vi "Framework Page.vi"(8 "error in (no error)":errorcluster, 11 "Node Ptr":T1 format="%.0x") -> (0 "error out":errorcluster)   [LabVIEW 2017, in "DSF System Explorer.lvlib"]
uses:
  DSF System Explorer.lvlib
  <vilib>/NI Veristand/Custom Device API/Custom Device Item Ref.ctl
  <vilib>/NI Veristand/Custom Device API/Custom Device API.lvlib
  Shared/DSF Shared.lvlib
panel:
  in  "Launch Data Viewer":bool
  in  "Server Frequency":dbl=20.0 format="%.0f Hz"
  in  "Enable Data Server":bool
  in  "Show Dialog on Error":bool
  in  "Show Threads":bool
  in  "Infinite FIFO Timeouts":bool
  in  "Measure Durations":bool
  in  "Measure Period":bool
  in  "Refresh Configuration":bool
  in  "View Configuration":bool
  in  "DSF Configuration Path":path
  in  "Header":cluster{"Section Name":string}={"Section Name"="Data Sharing Framework"}
  # "Debug Options"
  # "Measurement Options"
  # "Data Server Options"
  # "All Targets"
  # "All Targets"
  # "All Targets"
  # "Windows Only"
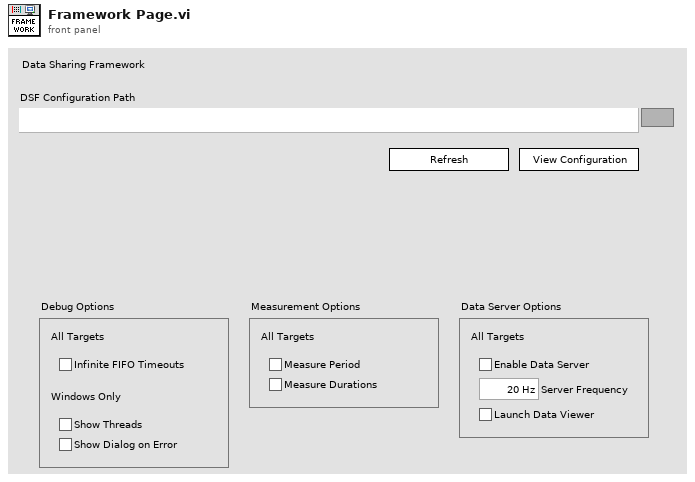
[diagram p1: front panel]
types:
  T1 = typedef "Custom Device API.lvlib/Custom Device Item Ref.ctl" = u64
  T2 = typedef "DSF Core.lvlibp/Framework.lvclass/Framework Options.ctl" = cluster{"FIFO Options":T3, "Thread Options":T4, "Plugin Options":T5, "Performance Options":T6, "Data Server Options":T7}
  T3 = typedef "DSF Core.lvlibp/Framework.lvclass/DSF FIFO Options.ctl" = cluster{"Infinite Timeouts":bool}
  T4 = typedef "DSF Core.lvlibp/Thread.lvclass/Thread Options.ctl" = cluster{"Show FP On Call":bool, "Close FP After Call":bool, "Allow Debugging":bool}
  T5 = typedef "DSF Core.lvlibp/Framework.lvclass/DSF Plugin Options.ctl" = cluster{"Default Components":bool}
  T6 = typedef "DSF Core.lvlibp/DSF Performance Options.ctl" = cluster{"Measure Period":bool, "Measure Rx/Tx Duration":bool}
  T7 = typedef "DSF Core.lvlibp/Framework.lvclass/Data Server Options.ctl" = cluster{"Enable Data Server":bool, "Period":u32}
  T8 = typedef "Custom Device API.lvlib/Custom Device Commands.ctl" = enum16{"Default", "Item renamed", "Shutdown", "Dynamic button pressed"}
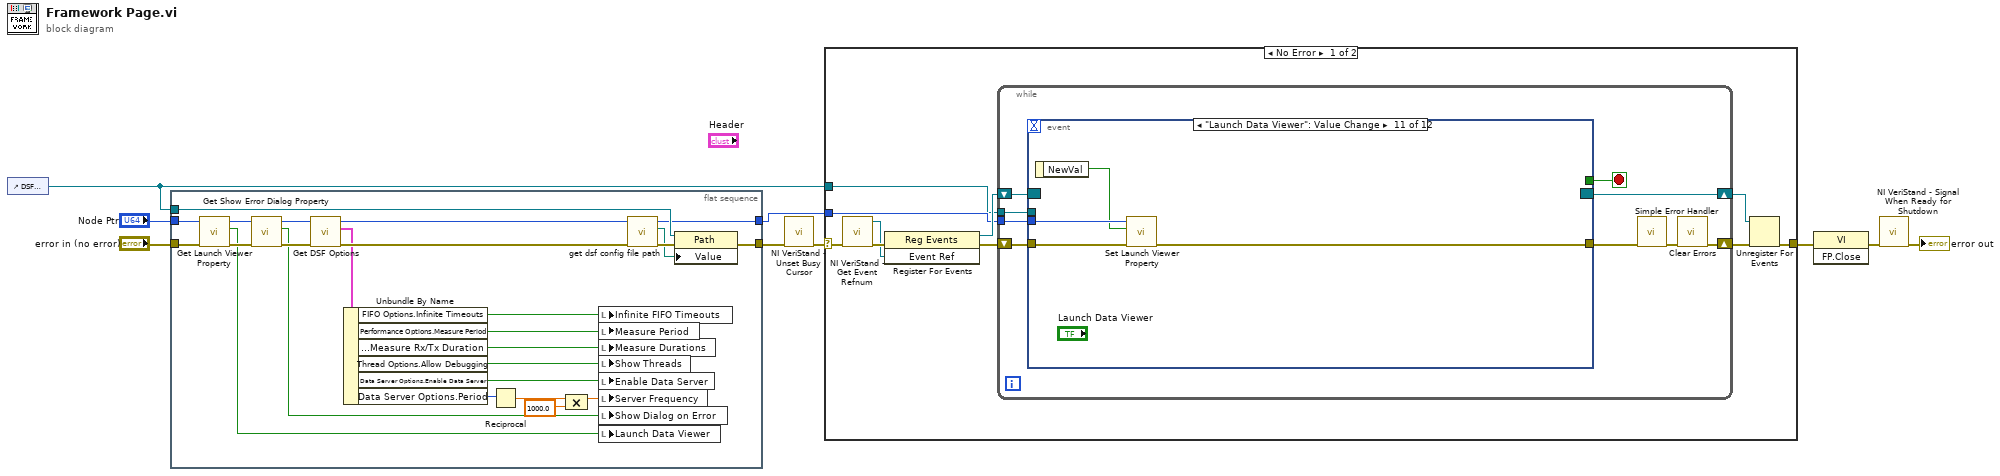
[diagram p0: block diagram]
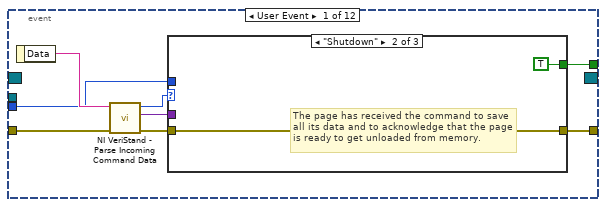
[diagram p2: hidden frame]
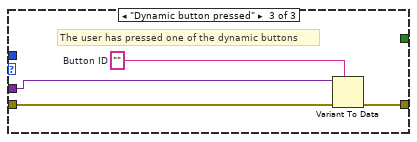
[diagram p4: hidden frame]
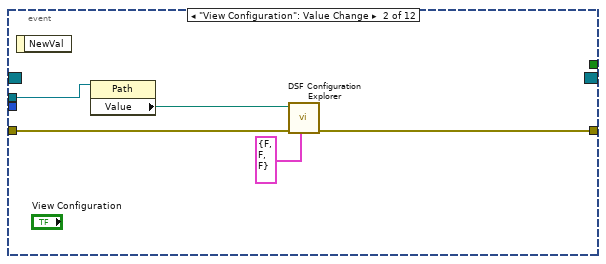
[diagram p5: hidden frame]
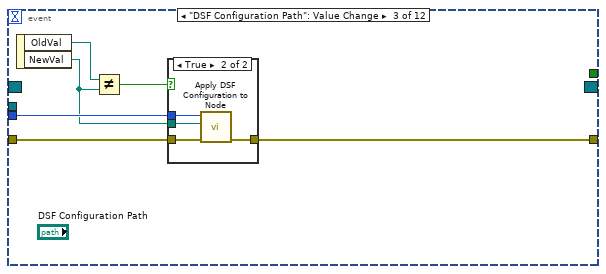
[diagram p6: hidden frame]
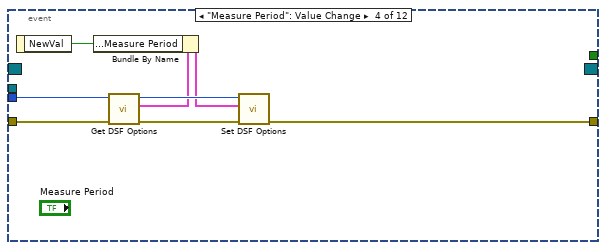
[diagram p8: hidden frame]
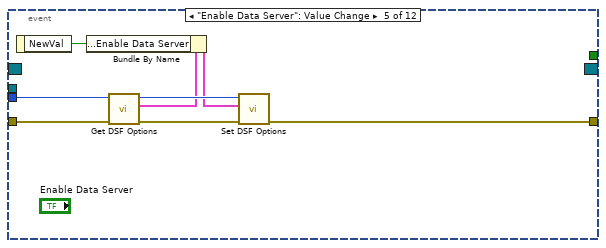
[diagram p9: hidden frame]
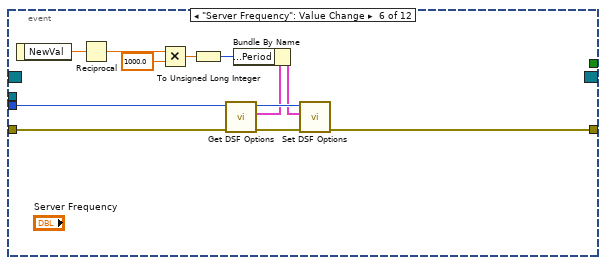
[diagram p10: hidden frame]
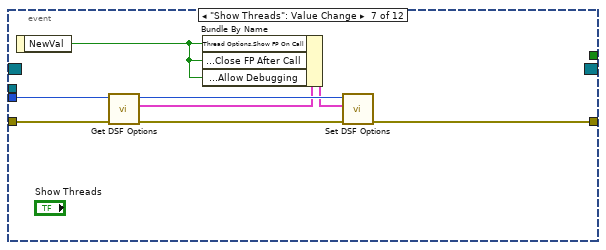
[diagram p11: hidden frame]
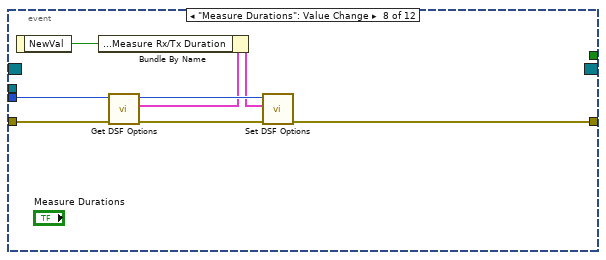
[diagram p12: hidden frame]
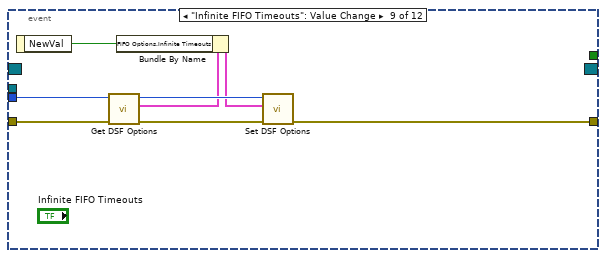
[diagram p13: hidden frame]
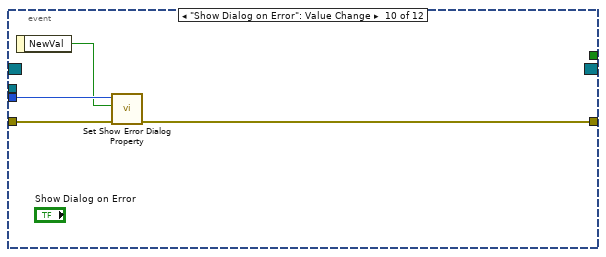
[diagram p14: hidden frame]
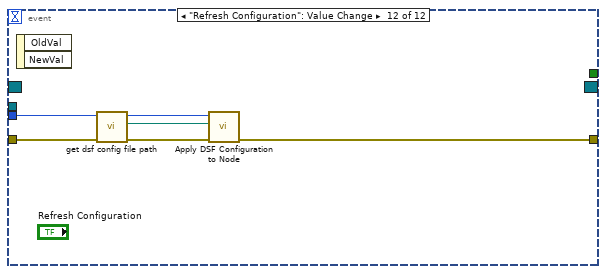
[diagram p15: hidden frame]
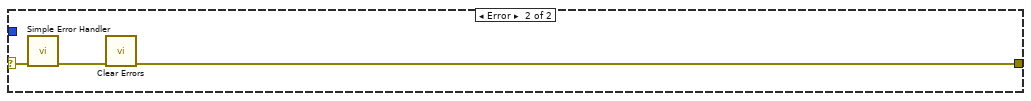
[diagram p16: hidden frame]
diagram:
  n1 = control-ref of="DSF Configuration Path"() -> (w1:refnum<vi>)
  n2 = flat-sequence "Initialization code" {
    tunnel: "error in (no error)" -> [w14]
    tunnel: "Node Ptr" -> [w13]
    tunnel: [w33] -> w5
    tunnel: [w31] -> w2
    tunnel: w1 -> [w32]
    frame #0 {
      n3 = call "Get Launch Viewer Property.vi"("error in (no error)"=w14, "Item Ref in"=w13) -> ("error out"=w12:errorcluster, "launch viewer"=w10:bool, "Item Ref out"=w11:T1)  [unwired: 7 in]
      n4 = call "Get Show Error Dialog Property.vi"("error in (no error)"=w12, "Item Ref in"=w11) -> ("error out"=w21:errorcluster, "show error dialog"=w15:bool, "Item Ref out"=w22:T1)  [unwired: 7 in]
      n5 = call "Get DSF Options.vi"("error in (no error)"=w21, "Item Ref in"=w22) -> ("error out"=w24:errorcluster, "options"=w23:T2, "Item Ref out"=w25:T1)  [unwired: 7 in]
      n6 = Unbundle By Name(w23) -> ("FIFO Options.Infinite Timeouts"=w29:bool, "Performance Options.Measure Period"=w28:bool, "Performance Options.Measure Rx/Tx Duration"=w27:bool, "Thread Options.Allow Debugging"=w26:bool, "Data Server Options.Enable Data Server"=w20:bool, "Data Server Options.Period"=w19:u32)
      n7 = Reciprocal(x=w19) -> (1/x=w18:dbl)
      n8 = Compound Arithmetic op=MULTIPLY(w18, 1000.0 ("y")) -> (w17:dbl)
      n9 = local write "Infinite FIFO Timeouts"(w29) -> ()
      n10 = local write "Measure Period"(w28) -> ()
      n11 = local write "Measure Durations"(w27) -> ()
      n12 = local write "Show Threads"(w26) -> ()
      n13 = local write "Enable Data Server"(w20) -> ()
      n14 = local write "Server Frequency"(w17) -> ()
      n15 = local write "Show Dialog on Error"(w15) -> ()
      n16 = local write "Launch Data Viewer"(w10) -> ()
      n17 = call "get dsf config file path.vi"("error in (no error)"=w24, "Node Ptr"=w25) -> ("error out"=w34:errorcluster, "Path"=w30:path, "Item Ref out"=w31:T1)  [unwired: 6 in, 1 out]
      n18 = property class="Path"(reference=w32, error in=w34, "Value"=w30) -> (error out=w33:errorcluster)  [unwired: 1 out]
    }
  }
  n19 = call <vilib>:"NI VeriStand - Unset Busy Cursor.vi"("error in (no error)"=w5) -> ("error out"=w4:errorcluster)  [unwired: 10 out]
  n20 = case shown="No Error" w4 {
    selector: w4 -> [w36 w153]
    tunnel: [w41 w151] -> w9
    tunnel: w2 -> [w37 _]
    tunnel: w1 -> [w35 _]
    frame No Error {
      n21 = call <vilib>:"NI VeriStand - Get Event Refnum.vi"("error in (no error)"=w36) -> ("error out"=w44:errorcluster, "Event Ref"=w40:refnum<user-event>)  [unwired: 9 out]
      n22 = register-events(error in=w44, w40) -> (reference out=w38:refnum<event-registration>, error out=w39:errorcluster)  [unwired: 1 in]
      n23 = while {
        tunnel: w37 -> [w49]
        shift-right: [w46] -> w42
        shift-left: w39 -> [w52]
        shift-right: [w53] -> w43
        shift-left: w38 -> [w51]
        tunnel: w35 -> [w45]
        stop <- w50 stop-if-true
        n24 = event shown="[10] \"Launch Data Viewer\": Value Change" {
          selector: w51 -> [_ _ _ _ _ _ _ _ _ _ _ _]
          dyn-events: [_ _ _ _ _ _ _ _ _ _ _ _] -> w53
          timeout: _ -> [_ _ _ _ _ _ _ _ _ _ _ _]
          tunnel: w52 -> [w61 w73 w79 w90 w98 w111 w119 w126 w134 w140 w144 w150]
          tunnel: [w57 _ _ _ _ _ _ _ _ _ _ _] -> w50
          tunnel: [w56 w72 w77 w87 w95 w109 w116 w123 w131 w138 w143 w145] -> w48
          tunnel: w49 -> [w55 _ w78 w92 w100 w112 w120 w128 w136 w139 w142 w148]
          tunnel: w45 -> [_ w71 _ _ _ _ _ _ _ _ _ _]
          event User Event {
            n25 = event-data() -> ("Data"=w60:string)  [unwired: 1 out]
            n26 = call <vilib>:"NI VeriStand - Parse Incoming Command Data.vi"("error in (no error)"=w61, "Incoming data"=w60) -> ("error out"=w59:errorcluster, "Outgoing data"=w54:variant, "Action"=w58:T8)  [unwired: 7 out]
            n27 = case shown="\"Shutdown\"" w58 {
              tunnel: w59 -> [w62 w63 w68]
              tunnel: [_ TRUE _] -> w57
              tunnel: [w62 w63 w65] -> w56
              tunnel: w55 -> [_ _ _]
              tunnel: w54 -> [_ _ w67]
              frame "Default", Default {
              }
              frame "Shutdown" {
                # "The page has received the command to save all its data and to acknowledge that the page is ready to get unloaded from memory."
              }
              frame "Dynamic button pressed" {
                w66 = ""  # Button ID
                # "The user has pressed one of the dynamic buttons"
                n28 = Variant To Data(error in=w68, type=w66, Variant=w67) -> (error out=w65:errorcluster)  [unwired: 1 out]
              }
            }
          }
          event "View Configuration": Value Change {
            n29 = event-data() -> ()  [unwired: 2 out]
            n30 = property class="Path"(reference=w71) -> ("Value"=w70:path)  [unwired: 1 in, 2 out]
            n31 = call "DSF Configuration Explorer.vi"("menu options"=cluster{"open":bool, "save":bool, "view":bool} {"open"=FALSE, "save"=FALSE, "view"=FALSE}, "error in (no error)"=w73, "Path in"=w70) -> ("error out"=w72:errorcluster)  [unwired: 7 in, 1 out]
          }
          event "DSF Configuration Path": Value Change {
            n32 = event-data() -> ("OldVal"=w76:path, "NewVal"=w75:path)  [unwired: 1 out]
            n33 = Not Equal?(x=w76, y=w75) -> (x != y?=w74:bool)
            n34 = case shown="True" w74 {
              tunnel: w79 -> [w80 w84]
              tunnel: w78 -> [_ w81]
              tunnel: [w80 w83] -> w77
              tunnel: w75 -> [_ w82]
              frame False {
              }
              frame True {
                n35 = call "Apply DSF Configuration to Node.vi"("error in (no error)"=w84, "NewVal"=w82, "Item Ref in"=w81) -> ("error out"=w83:errorcluster)  [unwired: 8 in]
              }
            }
          }
          event "Measure Period": Value Change {
            n36 = event-data() -> ("NewVal"=w91:bool)  [unwired: 1 out]
            n37 = call "Get DSF Options.vi"("error in (no error)"=w90, "Item Ref in"=w92) -> ("error out"=w88:errorcluster, "options"=w85:T2, "Item Ref out"=w89:T1)  [unwired: 7 in]
            n38 = Bundle By Name(cluster=w85, "Performance Options.Measure Period"=w91) -> (w86:T2)
            n39 = call "Set DSF Options.vi"("error in (no error)"=w88, "options"=w86, "Item Ref in"=w89) -> ("error out"=w87:errorcluster)  [unwired: 7 in, 1 out]
          }
          event "Enable Data Server": Value Change {
            n40 = event-data() -> ("NewVal"=w99:bool)  [unwired: 1 out]
            n41 = call "Get DSF Options.vi"("error in (no error)"=w98, "Item Ref in"=w100) -> ("error out"=w96:errorcluster, "options"=w93:T2, "Item Ref out"=w97:T1)  [unwired: 7 in]
            n42 = Bundle By Name(cluster=w93, "Data Server Options.Enable Data Server"=w99) -> (w94:T2)
            n43 = call "Set DSF Options.vi"("error in (no error)"=w96, "options"=w94, "Item Ref in"=w97) -> ("error out"=w95:errorcluster)  [unwired: 7 in, 1 out]
          }
          event "Server Frequency": Value Change {
            n44 = event-data() -> ("NewVal"=w106:dbl)  [unwired: 1 out]
            n45 = Reciprocal(x=w106) -> (1/x=w102:dbl)
            n46 = Multiply(x=w102, y=1000.0) -> (x*y=w103:dbl)
            n47 = To Unsigned Long Integer(number=w103) -> (unsigned 32bit integer=w105:u32)
            n48 = call "Get DSF Options.vi"("error in (no error)"=w111, "Item Ref in"=w112) -> ("error out"=w104:errorcluster, "options"=w107:T2, "Item Ref out"=w110:T1)  [unwired: 7 in]
            n49 = Bundle By Name(cluster=w107, "Data Server Options.Period"=w105) -> (w108:T2)
            n50 = call "Set DSF Options.vi"("error in (no error)"=w104, "options"=w108, "Item Ref in"=w110) -> ("error out"=w109:errorcluster)  [unwired: 7 in, 1 out]
          }
          event "Show Threads": Value Change {
            n51 = event-data() -> ("NewVal"=w113:bool)  [unwired: 1 out]
            n52 = call "Get DSF Options.vi"("error in (no error)"=w119, "Item Ref in"=w120) -> ("error out"=w117:errorcluster, "options"=w114:T2, "Item Ref out"=w118:T1)  [unwired: 7 in]
            n53 = Bundle By Name(cluster=w114, "Thread Options.Show FP On Call"=w113, "Thread Options.Close FP After Call"=w113, "Thread Options.Allow Debugging"=w113) -> (w115:T2)
            n54 = call "Set DSF Options.vi"("error in (no error)"=w117, "options"=w115, "Item Ref in"=w118) -> ("error out"=w116:errorcluster)  [unwired: 7 in, 1 out]
          }
          event "Measure Durations": Value Change {
            n55 = event-data() -> ("NewVal"=w127:bool)  [unwired: 1 out]
            n56 = call "Get DSF Options.vi"("error in (no error)"=w126, "Item Ref in"=w128) -> ("error out"=w124:errorcluster, "options"=w121:T2, "Item Ref out"=w125:T1)  [unwired: 7 in]
            n57 = Bundle By Name(cluster=w121, "Performance Options.Measure Rx/Tx Duration"=w127) -> (w122:T2)
            n58 = call "Set DSF Options.vi"("error in (no error)"=w124, "options"=w122, "Item Ref in"=w125) -> ("error out"=w123:errorcluster)  [unwired: 7 in, 1 out]
          }
          event "Infinite FIFO Timeouts": Value Change {
            n59 = event-data() -> ("NewVal"=w135:bool)  [unwired: 1 out]
            n60 = call "Get DSF Options.vi"("error in (no error)"=w134, "Item Ref in"=w136) -> ("error out"=w132:errorcluster, "options"=w129:T2, "Item Ref out"=w133:T1)  [unwired: 7 in]
            n61 = Bundle By Name(cluster=w129, "FIFO Options.Infinite Timeouts"=w135) -> (w130:T2)
            n62 = call "Set DSF Options.vi"("error in (no error)"=w132, "options"=w130, "Item Ref in"=w133) -> ("error out"=w131:errorcluster)  [unwired: 7 in, 1 out]
          }
          event "Show Dialog on Error": Value Change {
            n63 = event-data() -> ("NewVal"=w137:bool)  [unwired: 1 out]
            n64 = call "Set Show Error Dialog Property.vi"("error in (no error)"=w140, "show error dialog"=w137, "Item Ref in"=w139) -> ("error out"=w138:errorcluster)  [unwired: 7 in, 1 out]
          }
          event "Launch Data Viewer": Value Change {
            n65 = event-data() -> ("NewVal"=w141:bool)  [unwired: 1 out]
            n66 = call "Set Launch Viewer Property.vi"("error in (no error)"=w144, "launch viewer"=w141, "Item Ref in"=w142) -> ("error out"=w143:errorcluster)  [unwired: 7 in, 1 out]
          }
          event "Refresh Configuration": Value Change {
            n67 = event-data() -> ()  [unwired: 3 out]
            n68 = call "get dsf config file path.vi"("error in (no error)"=w150, "Node Ptr"=w148) -> ("error out"=w149:errorcluster, "Path"=w146:path, "Item Ref out"=w147:T1)  [unwired: 6 in, 1 out]
            n69 = call "Apply DSF Configuration to Node.vi"("error in (no error)"=w149, "NewVal"=w146, "Item Ref in"=w147) -> ("error out"=w145:errorcluster)  [unwired: 8 in]
          }
        }
        n70 = call <vilib>:"Simple Error Handler.vi"("error in (no error)"=w48) -> ("error out"=w47:errorcluster)  [unwired: 1 in, 7 out]
        n71 = call <vilib>:"Clear Errors.vi"("error in (no error)"=w47) -> ("error out"=w46:errorcluster)  [unwired: 1 in, 5 out]
      }
      n72 = Unregister For Events(event registration refnum=w43, error in=w42) -> (error out=w41:errorcluster)
    }
    frame Error {
      n73 = call <vilib>:"Simple Error Handler.vi"("error in (no error)"=w153) -> ("error out"=w152:errorcluster)  [unwired: 1 in, 7 out]
      n74 = call <vilib>:"Clear Errors.vi"("error in (no error)"=w152) -> ("error out"=w151:errorcluster)  [unwired: 1 in, 5 out]
    }
  }
  n75 = invoke class="VI" method="FP.Close"(error in=w9) -> (error out=w8:errorcluster)  [unwired: 2 in, 2 out]
  n76 = call <vilib>:"NI VeriStand - Signal When Ready for Shutdown.vi"("error in (no error)"=w8) -> ("error out"=→"error out":errorcluster)  [unwired: 10 out]
